vi "Teleop.vi"(10 "Match Info":T1={"Autonomous Elapsed Seconds"=0.0, "TeleOp Elapsed Seconds"=0.0, "Disabled Elapsed Seconds"=0.0, "Visited Autonomous"=FALSE, "Visited TeleOp"=FALSE, "Visited Disabled"=FALSE, "Autonomous Settings"={"Autonomous Style"=enum."Independent", "VI Refnum"=refnum}}, 11 "Call Context":T2) -> ()   [LabVIEW 2018]
doc: "This VI is called for each TeleOp packet received from the DS where the robot is not disabled. It is often used to read from the joysticks and update I/O or to update setpoints for timed control loops. It should complete and return within 20 milliseconds or it may miss DS packets."
uses:
  <vilib>/Rock Robotics/WPI/DriverStation/WPI_DriverStationDerivedRobotMode.ctl
  <vilib>/Rock Robotics/WPI/DriverStation/WPI_DriverStationMatch Info.ctl
  <vilib>/Rock Robotics/WPI/Utilities/WPI_GetSetVariantRefNum.vi
  Robot Global Data.vi
  <vilib>/Rock Robotics/Network Tables/NT Write Boolean Array.vi
  <vilib>/Rock Robotics/Network Tables/NT Write Numeric Array.vi
  <vilib>/Rock Robotics/Network Tables/NT Read Boolean.vi
  <vilib>/Rock Robotics/Network Tables/NT Read Number.vi
panel:
  out "Sample Slider 0":dbl(slide) scale=0.0..5.0
  out "Sample Boolean 1":bool
  out "Sample Boolean 0":bool
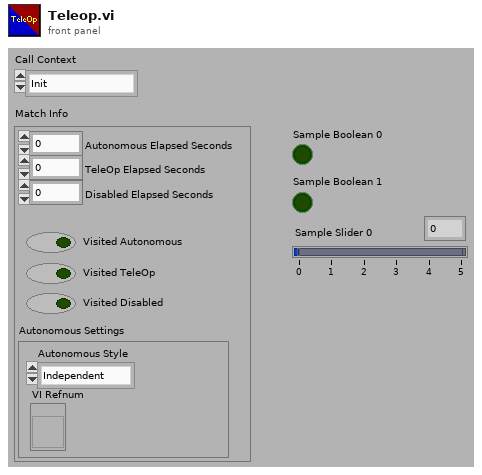
[diagram p1: front panel]
types:
  T1 = typedef "WPI_DriverStationMatch Info.ctl" = cluster{"Autonomous Elapsed Seconds":dbl, "TeleOp Elapsed Seconds":dbl, "Disabled Elapsed Seconds":dbl, "Visited Autonomous":bool, "Visited TeleOp":bool, "Visited Disabled":bool, "Autonomous Settings":cluster{"Autonomous Style":enum16{"Iterative", "Independent"}, "VI Refnum":refnum<vi>}}
  T2 = typedef "WPI_DriverStationDerivedRobotMode.ctl" = enum16{"Init", "Execute", "Stop"}
  T3 = typedef "WPI_JoystickDevRef.ctl" = cluster{"Device":T4}
  T4 = typedef "WPI_JoystickDeviceEnum.ctl" = enum16{"USB 0", "USB 1", "USB 2", "USB 3", "USB 4", "USB 5"}
  T5 = typedef "WPI_RobotDriveDevRef.ctl" = cluster{"DevStatus":errorcluster, "Motors[]":T6[], "Square Inputs":bool, "Max Output":dbl}
  T6 = typedef "WPI_MotorControlDeviceRef.ctl" = cluster{"DeviceStatus":errorcluster, "Type":T7, "PWM":cluster{"PWM Channel":T8, "DeadBand":T9}, "CAN":cluster{"Device Number":u8, "SetOutput VI Ref":variant, "GetOutput VI Ref":variant, "Enable VI Ref":variant, "Disable VI Ref":variant, "Data":variant}, "Invert":bool, "DIO PWM":cluster{"PWM \"Enable\" Channel":T8, "DIOChannel":T10, "PWM Rate":dbl}}
  T7 = typedef "WPI_MotorControlType.ctl" = enum16{"PWM", "CAN", "DIO PWM"}
  T8 = typedef "FPGA_DIOPWMChannel.ctl" = enum8{"PWM 0", "PWM 1", "PWM 2", "PWM 3", "PWM 4", "PWM 5", "PWM 6", "PWM 7", "PWM 8", "PWM 9", "PWM MXP 0", "PWM MXP 1", "PWM MXP 2", "PWM MXP 3", "PWM MXP 4", "PWM MXP 5", "PWM MXP 6", "PWM MXP 7", "PWM MXP 8", "PWM MXP 9", "Invalid"}
  T9 = typedef "WPI_PWMDeadband.ctl" = cluster{"Name":string, "maxPositivePwm":i32, "minPositivePwm":i32, "centerPwm":i32, "maxNegativePwm":i32, "minNegativePwm":i32, "angularRange":u16}
  T10 = typedef "FPGA_DIOChannel.ctl" = enum8{"DIO 0", "DIO 1", "DIO 2", "DIO 3", "DIO 4", "DIO 5", "DIO 6", "DIO 7", "DIO 8", "DIO 9", "DIO MXP 0", "DIO MXP 1", "DIO MXP 2", "DIO MXP 3", "DIO MXP 4", "DIO MXP 5", "DIO MXP 6", "DIO MXP 7", "DIO MXP 8", "DIO MXP 9", "DIO MXP 10", "DIO MXP 11", "DIO MXP 12", "DIO MXP 13", "DIO MXP 14", "DIO MXP 15", "SPI Port CS1", "SPI Port CS2", "SPI Port CS3", "SPI Port MISO", "SPI Port MOSI", "Invalid"}
  T11 = cluster{"Axes[0]":dbl, "Axes[1]":dbl, "Axes[2]":dbl, "Axes[3]":dbl, "Axes[4]":dbl, "Axes[5]":dbl, "Axes[6]":dbl, "Axes[7]":dbl, "Axes[8]":dbl}
  T12 = cluster{"Buttons[0]":bool, "Buttons[1]":bool, "Buttons[2]":bool, "Buttons[3]":bool, "Buttons[4]":bool, "Buttons[5]":bool, "Buttons[6]":bool, "Buttons[7]":bool, "Buttons[8]":bool, "Buttons[9]":bool, "Buttons[10]":bool}
  T13 = cluster{"Buttons[0]":bool, "Buttons[1]":bool, "Buttons[2]":bool, "Buttons[3]":bool, "Buttons[4]":bool, "Buttons[5]":bool, "Buttons[6]":bool, "Buttons[7]":bool, "Buttons[8]":bool}
  T14 = typedef "ElevatorAndShift2.ctl" = cluster{"Drive Shift":bool, "Ground":bool, "Hatch Low":bool, "Hatch Mid":bool, "Hatch High":bool, "Cargo Low":bool, "Cargo Mid":bool, "Cargo High":bool, "Cargo Ship":bool, "Cargo Feed":bool}
  T15 = enum16{"Idle", "Ground", "Hatch Low", "Hatch Mid", "Hatch High", "Cargo Low", "Cargo Mid", "Cargo High", "Cargo Ship", "Cargo Feed"}
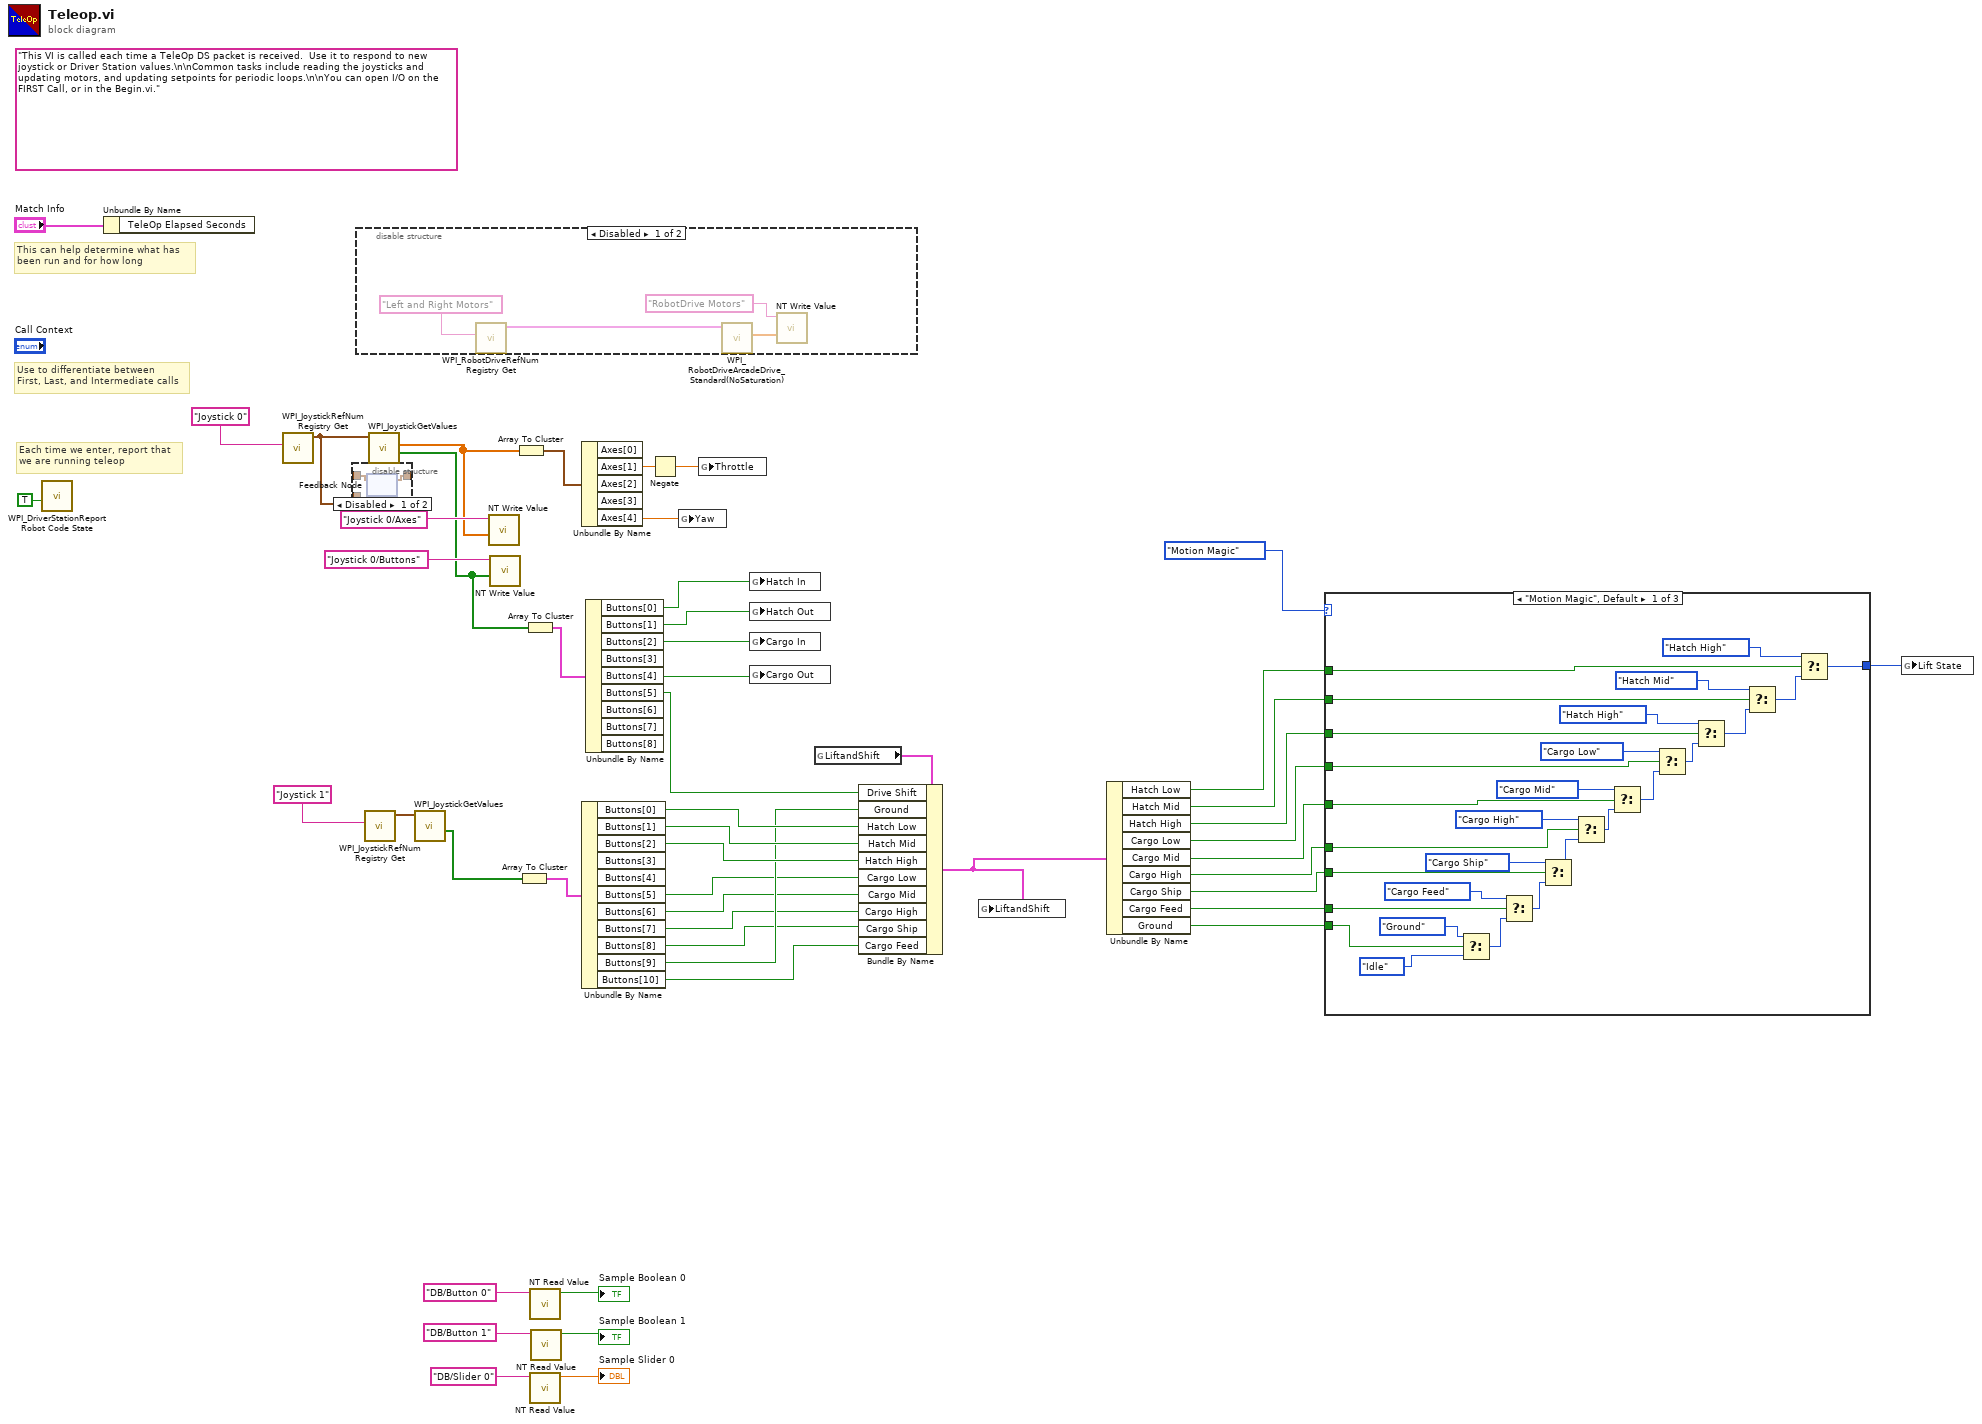
[diagram p0: block diagram]
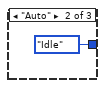
[diagram p2: hidden frame]
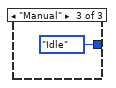
[diagram p3: hidden frame]
diagram:
  (unwired) "This VI is called each time a TeleOp DS packet is received.  Use it to respond to new joystick or Driver Station values.\n\nCommon tasks include reading the joysticks and updating motors, and updating setpoints for periodic loops.\n\nYou can open I/O on the FIRST Call, or in the Begin.vi."
  # "Each time we enter, report that\nwe are running teleop"
  # "Use to differentiate between\nFirst, Last, and Intermediate calls"
  # "This can help determine what has\nbeen run and for how long"
  n1 = call <vilib>:"WPI_DriverStationReport Robot Code State.vi"("TeleOp"=TRUE ("Autonomous")) -> ()  [unwired: 10 in, 1 out]
  n2 = Unbundle By Name("Match Info") -> ()  [unwired: 1 out]
  n3 = call <vilib>:"WPI_JoystickRefNum Registry Get.vi"("refnum name"="Joystick 0") -> ("JoystickDevRef"=w13:T3)  [unwired: 1 in, 9 out]
  n4 = disable-structure shown="Disabled" {
    disable-tunnel: _ -> [w53 _]
    disable-tunnel: [w52 _] -> _
    disable-tunnel: w13 -> [w51 _]
    frame Disabled {
      n5 = feedback #1(w51) -> (w52:T3)
      n6 = feedback-in #1(w53) -> ()
    }
    frame Enabled {
    }
  }
  n7 = disable-structure shown="Disabled" {
    frame Disabled {
      n8 = call <vilib>:"WPI_RobotDriveRefNum Registry Get.vi"("refnum name"="Left and Right Motors") -> ("RobotDriveDevRef"=w56:T5)  [unwired: 1 in, 9 out]
      n9 = call <vilib>:"WPI_RobotDriveArcadeDrive_Standard(NoSaturation).vi"("RobotDriveDevRef"=w56) -> ("Motor Values"=w54:dbl[])  [unwired: 3 in, 7 out]
      n10 = call-poly <vilib>:"NT Write Value.vi"("Numeric Array"=w54, "Name"="RobotDrive Motors") -> ()  [unwired: 9 in, 1 out]
    }
    frame Enabled {
    }
  }
  n11 = call <vilib>:"WPI_JoystickRefNum Registry Get.vi"("refnum name"="Joystick 1") -> ("JoystickDevRef"=w33:T3)  [unwired: 1 in, 9 out]
  n12 = call <vilib>:"WPI_JoystickGetValues.vi"("JoystickDevRef"=w13) -> ("Buttons"=w37:bool[], "Axes"=w39:dbl[])  [unwired: 6 in, 3 out]
  n13 = call <vilib>:"WPI_JoystickGetValues.vi"("JoystickDevRef"=w33) -> ("Buttons"=w34:bool[])  [unwired: 6 in, 4 out]
  n14 = call-poly <vilib>:"NT Write Value.vi"("Numeric Array"=w39, "Name"="Joystick 0/Axes") -> ()  [unwired: 9 in, 1 out]
  n15 = call-poly <vilib>:"NT Write Value.vi"("Boolean Array"=w37, "Name"="Joystick 0/Buttons") -> ()  [unwired: 9 in, 1 out]
  n16 = Array To Cluster(array=w39) -> (cluster=w38:T11)
  n17 = Array To Cluster(array=w34) -> (cluster=w35:T12)
  n18 = Array To Cluster(array=w37) -> (cluster=w36:T13)
  n19 = call-poly <vilib>:"NT Read Value.vi"("Name"="DB/Button 0" ("refnum name")) -> ("Boolean"=→"Sample Boolean 0":bool)  [unwired: 9 in, 1 out]
  n20 = call-poly <vilib>:"NT Read Value.vi"("Name"="DB/Slider 0" ("refnum name")) -> ("Numeric"=→"Sample Slider 0":dbl)  [unwired: 9 in, 1 out]
  n21 = call-poly <vilib>:"NT Read Value.vi"("Name"="DB/Button 1" ("refnum name")) -> ("Boolean"=→"Sample Boolean 1":bool)  [unwired: 9 in, 1 out]
  n22 = Unbundle By Name(w38) -> ("Axes[1]"=w15:dbl, "Axes[4]"=w16:dbl)  [unwired: 3 out]
  n23 = Unbundle By Name(w35) -> ("Buttons[0]"=w30:bool, "Buttons[1]"=w29:bool, "Buttons[2]"=w28:bool, "Buttons[5]"=w26:bool, "Buttons[6]"=w25:bool, "Buttons[7]"=w24:bool, "Buttons[8]"=w22:bool, "Buttons[9]"=w27:bool, "Buttons[10]"=w23:bool)  [unwired: 2 out]
  n24 = Unbundle By Name(w36) -> ("Buttons[0]"=w19:bool, "Buttons[1]"=w18:bool, "Buttons[2]"=w21:bool, "Buttons[3]"=w20:bool, "Buttons[5]"=w12:bool)  [unwired: 4 out]
  n25 = Negate(x=w15) -> (-x=w14:dbl)
  n26 = global write "Robot Global Data.vi" "Yaw"(w16) -> ()
  n27 = global write "Robot Global Data.vi" "Throttle"(w14) -> ()
  n28 = global write "Robot Global Data.vi" "Hatch In"(w19) -> ()
  n29 = global write "Robot Global Data.vi" "Hatch Out"(w18) -> ()
  n30 = global write "Robot Global Data.vi" "Cargo In"(w21) -> ()
  n31 = global write "Robot Global Data.vi" "Cargo Out"(w20) -> ()
  n32 = global read "Robot Global Data.vi" "LiftandShift"() -> (w31:T14)
  n33 = Bundle By Name(cluster=w31, "Drive Shift"=w12, "Ground"=w27, "Hatch Low"=w30, "Hatch Mid"=w29, "Hatch High"=w28, "Cargo Low"=w26, "Cargo Mid"=w25, "Cargo High"=w24, "Cargo Ship"=w22, "Cargo Feed"=w23) -> (w17:T14)
  n34 = global write "Robot Global Data.vi" "LiftandShift"(w17) -> ()
  n35 = Unbundle By Name(w17) -> ("Hatch Low"=w3:bool, "Hatch Mid"=w4:bool, "Hatch High"=w5:bool, "Cargo Low"=w6:bool, "Cargo Mid"=w7:bool, "Cargo High"=w8:bool, "Cargo Ship"=w9:bool, "Cargo Feed"=w10:bool, "Ground"=w2:bool)
  n36 = case shown="\"Motion Magic\", Default" enum16{"Motion Magic", "Auto", "Manual"}."Motion Magic" {
    tunnel: w10 -> [w84 _ _]
    tunnel: w9 -> [w81 _ _]
    tunnel: w8 -> [w78 _ _]
    tunnel: w7 -> [w75 _ _]
    tunnel: w6 -> [w72 _ _]
    tunnel: w5 -> [w70 _ _]
    tunnel: w4 -> [w65 _ _]
    tunnel: w3 -> [w64 _ _]
    tunnel: [w62 T15."Idle" ("t") T15."Idle" ("t")] -> w1
    tunnel: w2 -> [w60 _ _]
    frame "Motion Magic", Default {
      n37 = Select(t=T15."Ground", s=w60, f=T15."Idle") -> (s? t:f=w58:T15)
      n38 = Select(t=T15."Cargo Feed", s=w84, f=w58) -> (s? t:f=w82:T15)
      n39 = Select(t=T15."Cargo Ship", s=w81, f=w82) -> (s? t:f=w79:T15)
      n40 = Select(t=T15."Cargo High", s=w78, f=w79) -> (s? t:f=w76:T15)
      n41 = Select(t=T15."Cargo Mid", s=w75, f=w76) -> (s? t:f=w73:T15)
      n42 = Select(t=T15."Cargo Low", s=w72, f=w73) -> (s? t:f=w69:T15)
      n43 = Select(t=T15."Hatch High", s=w70, f=w69) -> (s? t:f=w66:T15)
      n44 = Select(t=T15."Hatch Mid", s=w65, f=w66) -> (s? t:f=w63:T15)
      n45 = Select(t=T15."Hatch High", s=w64, f=w63) -> (s? t:f=w62:T15)
    }
    frame "Auto" {
    }
    frame "Manual" {
    }
  }
  n46 = global write "Robot Global Data.vi" "Lift State"(w1) -> ()
